vi "FTW-Supervisor-LogEvent.vi"(0 "FTW Supervisor Connection":T1, 5 "Event Type":string, 7 "Event Data":string, 9 "Source (unwired for call chain)":string="CallChain", 11 "error in":errorcluster) -> (4 "FTW Supervisor Connection out":T1, 15 "error out":errorcluster)   [LabVIEW 2015]
uses:
  core/type/FTW-Type-Actor-Connector.ctl
  time/FTW-Time-RelativeTimer.vi
  error/FTW-ERR-ThrowError.vi
  reflection/FTW-Reflection-Type.vi
  error/FTW-ERR-NoErrorConstant.vi
  error/FTW-ERR-CallChain.vi
  string/FTW-STR-ReplaceWhitespace.vi
  reflection/FTW-Reflection-Array.vi
  reflection/FTW-Reflection-FTWObject.vi
  string/FTW-STR-Array-Delimit.vi
  lib/FTW-KernelFilepath.vi
  json/core/FTW-JSON-Core-EncodingFlags.vi
  codegen/xnode/json/fetch/FTW-JSON-Core-GetFlattenedValue.vi
  socket/support/FTW-Socket-Core-LibraryError.vi
  request/FTW-Request-InterpretResponse.vi
  codegen/xnode/FTW-Actor-Ask.xnode
  codegen/xnode/FTW-JSON-Fetch.xnode
panel:
  # "Inputs"
  # "Outputs"
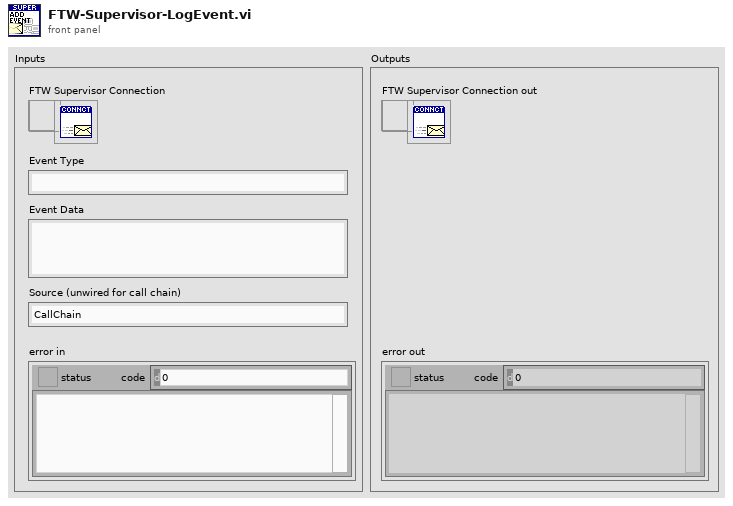
[diagram p1: front panel]
types:
  T1 = typedef "FTW-Type-Actor-Connector.ctl" = refnum<data-value>
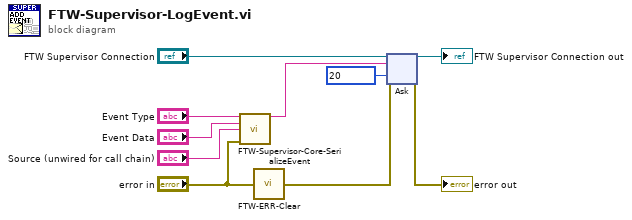
[diagram p0: block diagram]
diagram:
  n1 = call "FTW-Supervisor-Core-SerializeEvent.vi"("Event Type"="Event Type", "Event Data"="Event Data", "Source"="Source (unwired for call chain)", "Error to Log"="error in") -> ("Serialized Event"=w5:string)  [unwired: 11 in]
  n2 = call "FTW-ERR-Clear.vi"("error to snuff"="error in") -> ("no error"=w4:errorcluster)
  n3 = xnode "Ask"("FTW Actor Connector"="FTW Supervisor Connection", "Request"=w5, "Timeout"=20 ("Receive Timeout"), "error in"=w4) -> ("FTW Actor Connector out"=→"FTW Supervisor Connection out":T1, "error out"=→"error out":errorcluster)  [unwired: 1 in, 2 out]
